vi "Messages Test.vi"() -> ()   [LabVIEW 2019]
uses:
  simonMessages.lvclass
panel:
  in  "key":string="stageUp"
  out "Values":string
  in  "Messages Table":string[][](table)=[["welcome", "Welcome\r\nto\r\nLabVIEW Simon\r\nby\r\nFelipe Flores\r\n", "25", "Center", "LineByLine"], ["instructions", "\n\nSlide \"LEVEL\" to see how good you are.\n\nPress \"PLAY\" to start playing.\n\nPress \"LONGEST\" to see the longest sequence ever played.", "16", "Center", "Plain"], ["stageUp", "\\n\\rStage\\s%d", "60", "Center", "Rotate"], ["startGame", "\nLet's do it!", "40", "Center", "Plain"], ["last", "\nPlaying last Sequence...", "40", "Left", "Plain"], ["longest", "\nPlaying longest Sequence...", "40", "Left", "Plain"], ["hsHeaders", "High,Scores\r\n=========,=========\r\n", "25", "Center", "LineByLine"], ["levelChoice", "Level %d selected", "", "Left", "Plain"], ["yourTurn", "\n\nyour turn!", "40", "Center", "Plain"], ["gameTitle", "Simon Game", "10", "Left", "TitleBar"], ["playerName", "%s is playing now!", "10", "Left", "TitleBar"], ["", "", "", "", ""]]
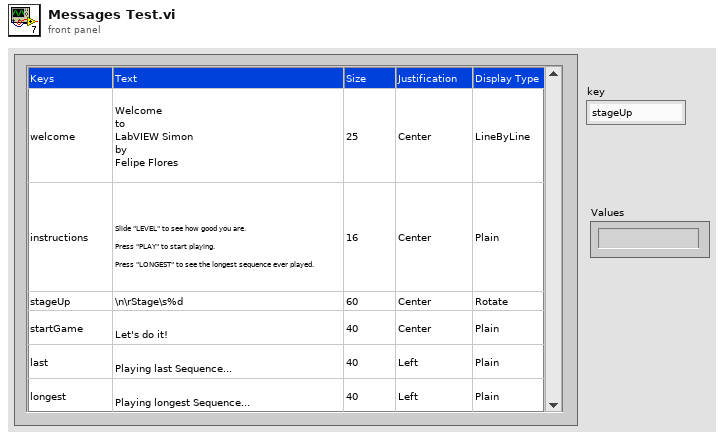
[diagram p1: front panel]
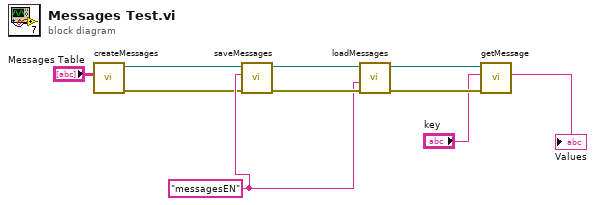
[diagram p0: block diagram]
diagram:
  w5 = "messagesEN" ("FileName (without extension)")
  n1 = call "createMessages.vi"("Messages Table"="Messages Table") -> ("error out"=w3:errorcluster, "simonMessages out"=w4:refnum<class "simonMessages.lvclass">)  [unwired: 9 in]
  n2 = call "saveMessages.vi"("error in (no error)"=w3, "FileName (without extension)"=w5, "simonMessages in"=w4) -> ("error out"=w10:errorcluster, "simonMessages out"=w7:refnum<class "simonMessages.lvclass">)  [unwired: 7 in]
  n3 = call "loadMessages.vi"("error in (no error)"=w10, "FileName (without extension)"=w5, "simonMessages in"=w7) -> ("error out"=w8:errorcluster, "simonMessages out"=w9:refnum<class "simonMessages.lvclass">)  [unwired: 7 in]
  n4 = call "getMessage.vi"("error in (no error)"=w8, "key"="key", "simonMessages in"=w9) -> ("Message Text"=→"Values":string)  [unwired: 6 in, 2 out]
